vi "Framework.Set Cache.vi"(10 "Cache":refnum<class "DSF.Engine.Memory.Cache.lvclass">, 11 "Framework in":refnum<class "Framework.lvclass">) -> (3 "Framework out":refnum<class "Framework.lvclass">)   [LabVIEW 2017, in "DSF.Engine.lvlib" / "Framework.lvclass"]
uses:
  Framework.lvclass
  Cache/DSF.Engine.Memory.Cache.lvclass
  Framework.lvclass/Framework.ctl
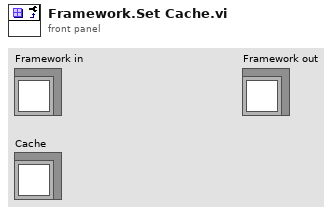
[diagram p1: front panel]
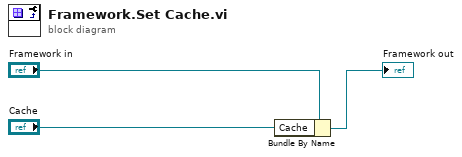
[diagram p0: block diagram]
diagram:
  n1 = Bundle By Name(cluster="Framework in", "Cache"="Cache") -> (→"Framework out":refnum<class "Framework.lvclass">)
